vi "ex_CorrectErrorChain.vi"(8 "error in (no error)":errorcluster, 10 "include warnings?":bool) -> (0 "error out":errorcluster)   [LabVIEW 2010]
doc: "Removes the first two items in this VI's call chain and makes that the source for the error out."
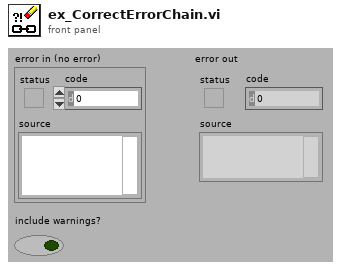
[diagram p1: front panel]
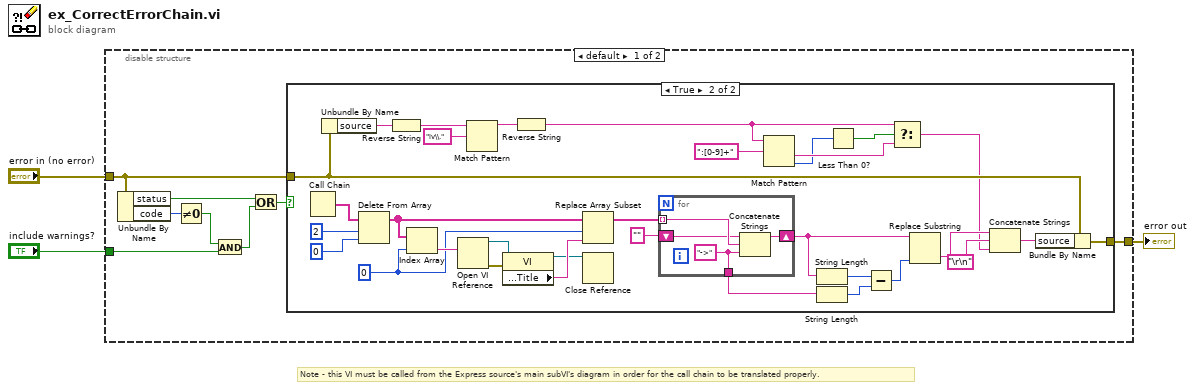
[diagram p0: block diagram]
diagram:
  # "Note - this VI must be called from the Express source's main subVI's diagram in order for the call chain to be translated properly."
  n1 = disable-structure shown="default" {
    disable-tunnel: [w11 w49] -> w3
    disable-tunnel: "error in (no error)" -> [w10 w49]
    disable-tunnel: "include warnings?" -> [w6 _]
    frame condition #0 (active) {
      n2 = Unbundle By Name(w10) -> ("status"=w8:bool, "code"=w7:i32)
      n3 = Not Equal To 0?(x=w7) -> (x != 0?=w5:bool)
      n4 = And(x=w5, y=w6) -> (x .and. y?=w4:bool)
      n5 = Or(x=w8, y=w4) -> (x .or. y?=w9:bool)
      n6 = case shown="True" w9 {
        tunnel: [w12 w44] -> w11
        tunnel: w10 -> [w12 w28]
        frame False {
        }
        frame True {
          w33 = 0 ("index")
          n7 = Call Chain() -> (call chain=w43:string[])
          n8 = Unbundle By Name(w28) -> ("source"=w27:string)
          n9 = Delete From Array(array=w43, length=2, index=0) -> (array with subset deleted=w35:string[])  [unwired: 1 out]
          n10 = Reverse String(1:w27) -> (0:w14:string)
          n11 = Index Array(array=w35, index=w33) -> (element=w37:string)
          n12 = Open VI Reference(vi path=w37) -> (vi reference=w40:refnum<vi>, error out=w39:errorcluster)  [unwired: 5 in]
          n13 = Match Pattern(string=w14, regular expression="iv\\.") -> (before substring=w24:string)  [unwired: 1 in, 3 out]
          n14 = property class="VI"(reference=w40, error in=w39) -> (reference out=w22:refnum<vi>, "Front Panel Window:Title"=w36:string)  [unwired: 1 out]
          n15 = Reverse String(1:w24) -> (0:w13:string)
          n16 = Replace Array Subset(array=w35, new element=w36, index=w33) -> (w34:string[])
          n17 = Close Reference(reference=w22) -> ()  [unwired: 1 in, 1 out]
          n18 = for {
            tunnel: w34 -> [w47] mode=indexing
            shift-right: [w48] -> w32
            shift-left: "" -> [w46]
            tunnel: [w45] -> w20
            w45 = "->" ("string")
            n19 = Concatenate Strings(w46, w47, w45) -> (w48:string)
          }
          n20 = Match Pattern(string=w13, regular expression=":[0-9]+") -> (after substring=w18:string, offset past match=w16:i32)  [unwired: 1 in, 2 out]
          n21 = String Length(string=w32) -> (length=w31:i32)
          n22 = String Length(string=w20) -> (length=w19:i32)
          n23 = Less Than 0?(x=w16) -> (x < 0?=w15:bool)
          n24 = Subtract(x=w31, y=w19) -> (x-y=w30:i32)
          n25 = Select(t=w13, s=w15, f=w18) -> (s? t:f=w17:string)
          n26 = Replace Substring(2:w30, 5:w32) -> (0:w29:string)  [unwired: 2 in, 1 out]
          n27 = Concatenate Strings(w29, "\r\n", w17) -> (w26:string)
          n28 = Bundle By Name(cluster=w28, "source"=w26) -> (w44:errorcluster)
        }
      }
    }
    frame condition #1 {
    }
  }
  "error out" <- w3
